vi "sub vi - cycle&temp fail v5.vi"(0 "Amps Lo?":bool, 2 "Input Cluster":T1, 3 "SELECT":T2(ring), 4 "Amps Hi?":bool, 5 "Result In":bool) -> (15 "(FAIL) out":cluster{"FAIL LO":dbl, "FAIL HI":dbl}, 16 "(DISP) out":T3, 17 "T-RISE":cluster{"T-RISE (L)":dbl, "T-RISE (N)":dbl}, 18 "Result Out":bool, 19 "file error":errorcluster)   [LabVIEW 2013]
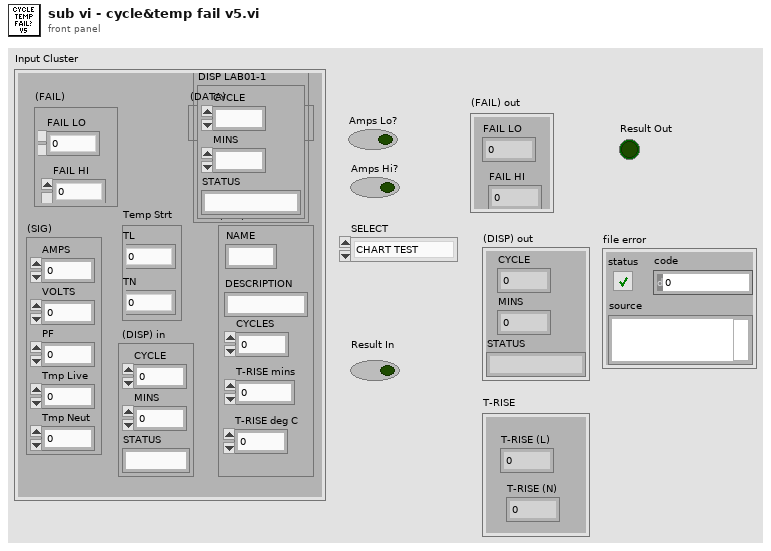
[diagram p1: front panel]
types:
  T1 = cluster{"(FAIL)":cluster{"FAIL LO":dbl, "FAIL HI":dbl}, "(SIG)":cluster{"AMPS":dbl, "VOLTS":dbl, "PF":dbl, "Tmp Live":dbl, "Tmp Neut":dbl}, "Temp Strt":cluster{"TL":dbl, "TN":dbl}, " (DISP) in":cluster{"CYCLE":dbl, "MINS":dbl, "STATUS":string}, "(SET)":cluster{"NAME":string, "DESCRIPTION":string, "CYCLES":dbl, "T-RISE mins":dbl, "T-RISE deg C":dbl}, "(DATA)":refnum<k1>}
  T2 = enum32{"CHART TEST", "CYCLE TEST", "T-RISE TEST"}
  T3 = cluster{"CYCLE":dbl, "MINS":dbl, "STATUS":string}
  T4 = cluster{"AMPS":dbl, "VOLTS":dbl, "PF":dbl, "Tmp Live":dbl, "Tmp Neut":dbl}
  T5 = cluster{"NAME":string, "DESCRIPTION":string, "CYCLES":dbl, "T-RISE mins":dbl, "T-RISE deg C":dbl}
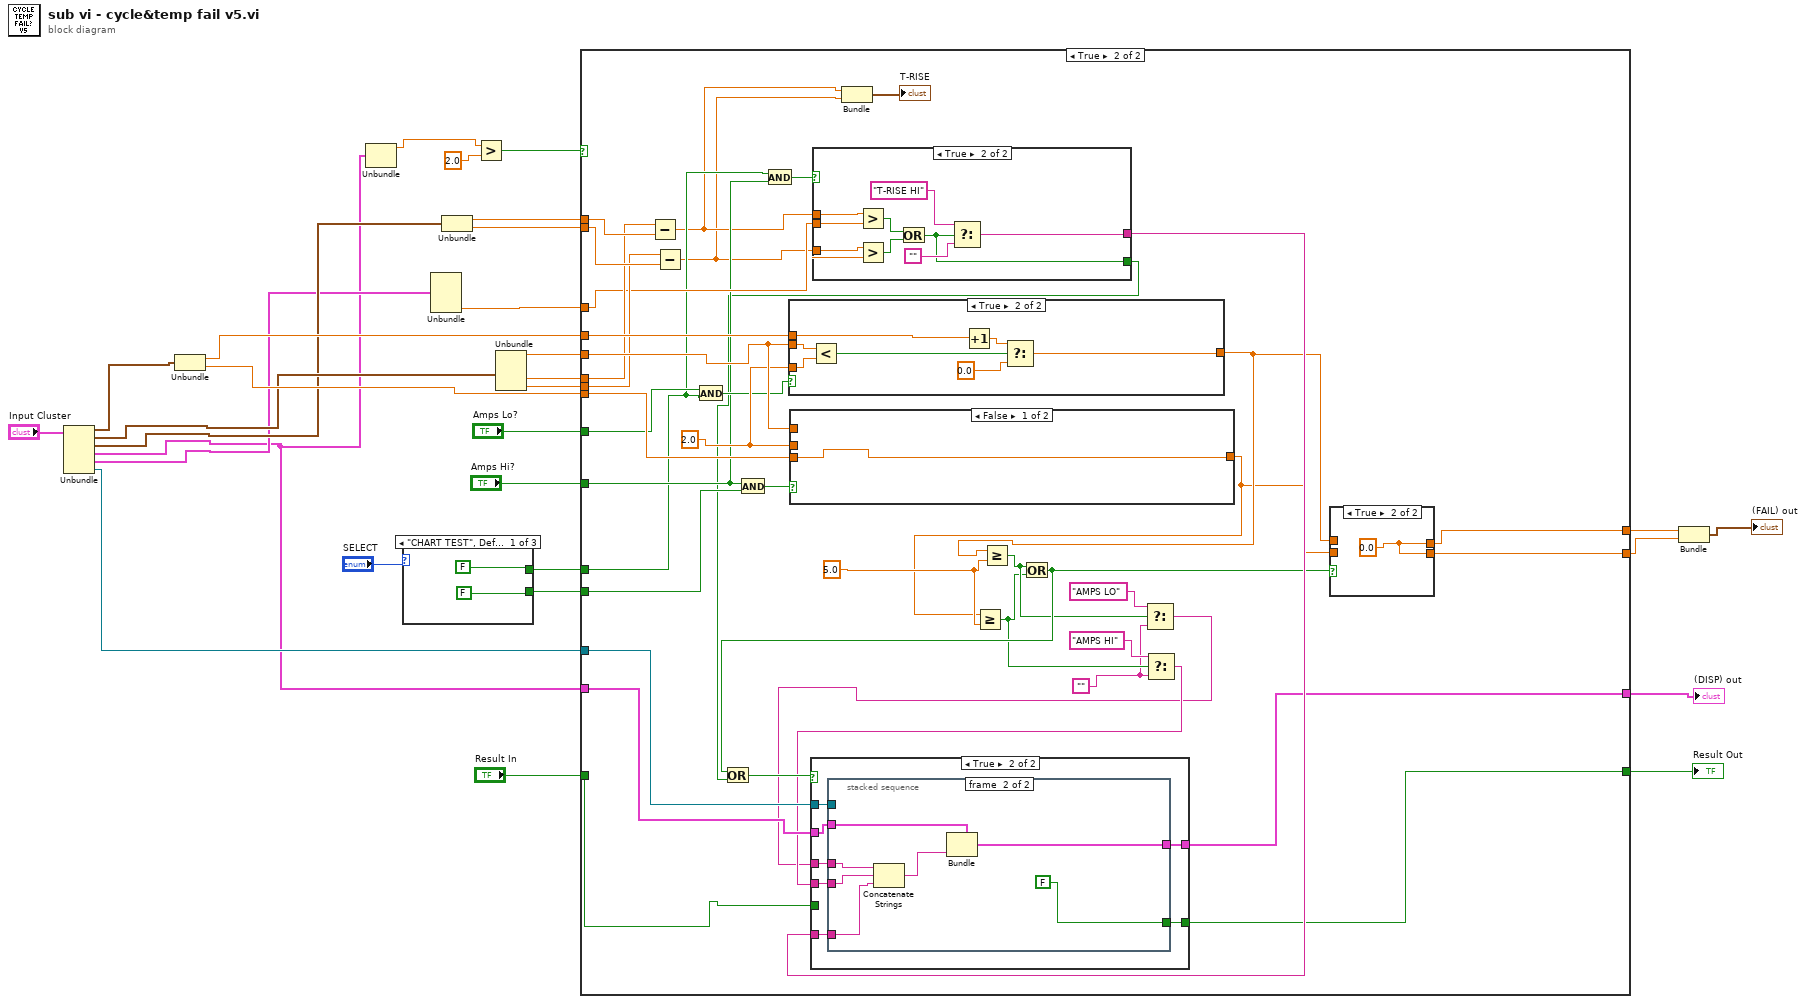
[diagram p0: block diagram]
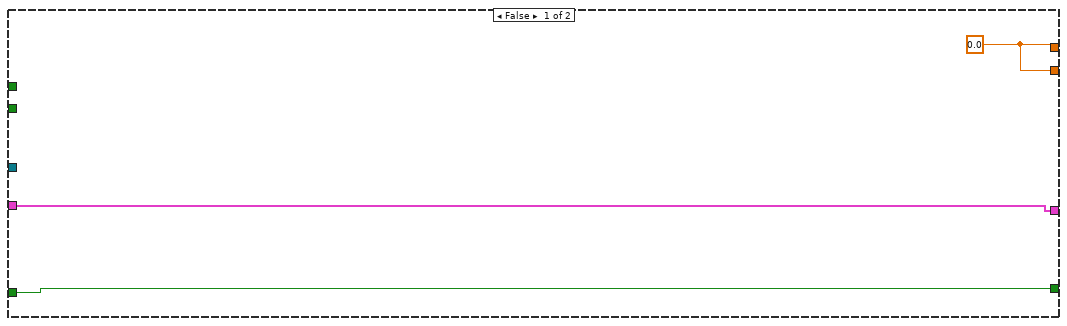
[diagram p2: hidden frame]
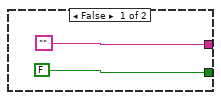
[diagram p4: hidden frame]
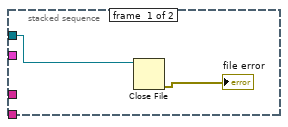
[diagram p6: hidden frame]
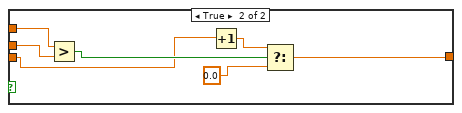
[diagram p7: hidden frame]
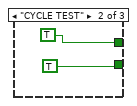
[diagram p9: hidden frame]
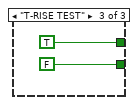
[diagram p10: hidden frame]
diagram:
  n1 = Unbundle("Input Cluster") -> ("(FAIL)"=w15:cluster{"FAIL LO":dbl, "FAIL HI":dbl}, "(SIG)"=w12:T4, "Temp Strt"=w11:cluster{"TL":dbl, "TN":dbl}, "(DISP) in"=w2:T3, "(SET)"=w10:T5, "(DATA)"=w9:refnum<k1>)
  n2 = Unbundle(w15) -> ("FAIL LO"=w14:dbl, "FAIL HI"=w13:dbl)
  n3 = Unbundle(w2) -> ("CYCLE"=w1:dbl)  [unwired: 2 out]
  n4 = case shown="\"CHART TEST\", Default" "SELECT" {
    tunnel: [FALSE TRUE TRUE] -> w19
    tunnel: [FALSE TRUE FALSE] -> w22
    frame "CHART TEST", Default {
    }
    frame "CYCLE TEST" {
    }
    frame "T-RISE TEST" {
    }
  }
  n5 = Unbundle(w10) -> ("T-RISE deg C"=w23:dbl)  [unwired: 4 out]
  n6 = Unbundle(w11) -> ("TL"=w27:dbl, "TN"=w26:dbl)
  n7 = Greater?(x=w1, y=2.0) -> (0:w17:bool)
  n8 = Unbundle(w12) -> ("AMPS"=w28:dbl, "Tmp Live"=w25:dbl, "Tmp Neut"=w24:dbl)  [unwired: 2 out]
  n9 = case shown="True" w17 {
    tunnel: w28 -> [_ w78]
    tunnel: w14 -> [_ w76]
    tunnel: w13 -> [_ w75]
    tunnel: w9 -> [_ w74]
    tunnel: w2 -> [w37 w73]
    tunnel: w27 -> [_ w72]
    tunnel: w26 -> [_ w71]
    tunnel: w25 -> [_ w70]
    tunnel: w24 -> [_ w69]
    tunnel: w23 -> [_ w68]
    tunnel: w22 -> [_ w64]
    tunnel: "Amps Lo?" -> [_ w62]
    tunnel: "Amps Hi?" -> [_ w60]
    tunnel: w19 -> [_ w59]
    tunnel: [w38 w56] -> w7
    tunnel: [w38 w55] -> w6
    tunnel: [w37 w54] -> w5
    tunnel: [w36 w53] -> w4
    tunnel: "Result In" -> [w36 w52]
    frame False {
      w38 = 0.0
    }
    frame True {
      w44 = ""
      w67 = 5.0
      w77 = 2.0
      n10 = Subtract(x=w70, y=w72) -> (x-y=w41:dbl)
      n11 = Subtract(x=w69, y=w71) -> (x-y=w40:dbl)
      n12 = And(x=w62, y=w59) -> (x .and. y?=w63:bool)
      n13 = And(x=w60, y=w64) -> (x .and. y?=w65:bool)
      n14 = And(x=w59, y=w60) -> (x .and. y?=w61:bool)
      n15 = case shown="True" w63 {
        tunnel: w78 -> [_ w126]
        tunnel: w77 -> [_ w125]
        tunnel: w76 -> [w119 w121]
        tunnel: [w119 w120] -> w58
        frame False {
        }
        frame True {
          n16 = Less?(x=w126, y=w125) -> (x < y?=w124:bool)
          n17 = Increment(x=w121) -> (x+1=w123:dbl)
          n18 = Select(t=w123, s=w124, f=0.0) -> (s? t:f=w120:dbl)
        }
      }
      n19 = case shown="False" w65 {
        tunnel: w78 -> [_ w118]
        tunnel: w77 -> [_ w117]
        tunnel: [w111 w113] -> w57
        tunnel: w75 -> [w111 w112]
        frame False {
        }
        frame True {
          n20 = Greater?(x=w118, y=w117) -> (0:w116:bool)
          n21 = Increment(x=w112) -> (x+1=w115:dbl)
          n22 = Select(t=w115, s=w116, f=0.0) -> (s? t:f=w113:dbl)
        }
      }
      n23 = case shown="True" w61 {
        tunnel: w68 -> [_ w92]
        tunnel: w41 -> [_ w85]
        tunnel: w40 -> [_ w84]
        tunnel: ["" w87] -> w66
        tunnel: [FALSE w86] -> w50
        frame False {
        }
        frame True {
          n24 = Greater?(x=w85, y=w92) -> (0:w90:bool)
          n25 = Greater?(x=w84, y=w92) -> (0:w91:bool)
          n26 = Or(x=w90, y=w91) -> (x .or. y?=w86:bool)
          n27 = Select(t="T-RISE HI", s=w86, f="") -> (s? t:f=w87:string)
        }
      }
      n28 = Bundle(w41, w40) -> (→"T-RISE":cluster{dbl, dbl})  [unwired: 1 in]
      n29 = Greater Or Equal?(x=w57, y=w67) -> (x >= y?=w47:bool)
      n30 = Greater Or Equal?(x=w58, y=w67) -> (x >= y?=w48:bool)
      n31 = Or(x=w48, y=w47) -> (x .or. y?=w51:bool)
      n32 = Or(x=w51, y=w50) -> (x .or. y?=w49:bool)
      n33 = Select(t="AMPS LO", s=w48, f=w44) -> (s? t:f=w42:string)
      n34 = Select(t="AMPS HI", s=w47, f=w44) -> (s? t:f=w43:string)
      n35 = case shown="True" w49 {
        tunnel: w42 -> [_ w101]
        tunnel: w43 -> [_ w100]
        tunnel: w73 -> [w94 w99]
        tunnel: w74 -> [_ w98]
        tunnel: w66 -> [_ w97]
        tunnel: [w94 w96] -> w54
        tunnel: [w93 w95] -> w53
        tunnel: w52 -> [w93 _]
        frame False {
        }
        frame True {
          n36 = stacked-sequence {
            tunnel: w101 -> [_ w110]
            tunnel: w100 -> [_ w109]
            tunnel: w99 -> [_ w107]
            tunnel: w98 -> [w103 _]
            tunnel: w97 -> [_ w106]
            tunnel: [_ w105] -> w96
            tunnel: [_ FALSE] -> w95
            frame #0 {
              n37 = Close File(refnum=w103) -> (error out=→"file error":errorcluster)  [unwired: 1 in, 1 out]
            }
            frame #1 {
              n38 = Concatenate Strings(w110, w109, w106) -> (w108:string)
              n39 = Bundle(cluster=w107, "STATUS"=w108) -> (w105:T3)  [unwired: 2 in]
            }
          }
        }
      }
      n40 = case shown="True" w51 {
        tunnel: w58 -> [w80 _]
        tunnel: w57 -> [w79 _]
        tunnel: [w80 w81] -> w56
        tunnel: [w79 w81] -> w55
        frame False {
        }
        frame True {
          w81 = 0.0
        }
      }
    }
  }
  "(DISP) out" <- w5
  "Result Out" <- w4
  n41 = Bundle("FAIL LO"=w7, "FAIL HI"=w6) -> (→"(FAIL) out":cluster{"FAIL LO":dbl, "FAIL HI":dbl})  [unwired: 1 in]
